vi "basic - VL Receive.vi"() -> ()   [LabVIEW 2020]
uses:
  _controls/comm_computedMAC-IP.ctl
  _controls/comm_verification_rx.ctl
  _controls/comm_udp_rx.ctl
  <extravilib>/ChannelInstances/Tag-bool/Write With Abort.vi
  <extravilib>/ChannelInstances/Tag-bool/Read With Abort.vi
  _polimorphicInstances/session/Fdx Create Session (Rx-VL-Oriented).vi
  bsp/AFDX_Receive/Fdx Create Rx VL.vi
  _polimorphicInstances/udpPort/Fdx Create UDP Port (RX-CommPort).vi
  _polimorphicInstances/control/Fdx Start (Rx).vi
  <extravilib>/ChannelInstances/Tag-bool/Instantiate.vi
  <extravilib>/ChannelInstances/Tag-bool/EndpointRead.vi
  <extravilib>/ChannelInstances/Tag-bool/Endpoint.vi
  _polimorphicInstances/control/Fdx Stop (Rx).vi
  _polimorphicInstances/session/Fdx Close Session (Port).vi
  AIM664LV.lvlib
  <extravilib>/ChannelInstances/Tag-bool.lvlib
panel:
  in  "DefaultPayloadMode (Full)":u32(ring) items=["FDX_PAYLOAD_FULL", "FDX_PAYLOAD_IP_EXT", "FDX_PAYLOAD_IP", "FDX_PAYLOAD_MAC"]
  in  "Board":u32
  in  "Port":u32=1
  out "CommPort Addresses":T1[](array[typedef])=[{"MACsrc"=[], "IPsrc"="10.1.33.1", "IPdest"="224.224.0.60"}, {"MACsrc"=[], "IPsrc"="10.1.33.1", "IPdest"="224.224.0.60"}] {"MACsrc" format="%.0x"}
  in  "VL Config":T2={"VlId"=60, "VLRange"=2, "VerificationMode"=0, "Bag"=0, "Jitter"=0, "MaxFrameLength"=0, "MaxSkew"=0, "VLBufSize"=32768, "FilterMode"=0, "FilterPosition"=0, "Padding"=0, "FilterMask"=0, "FilterData"=0, "MinFrameLength"=0} {"FilterMode" items=["FDX_RX_VL_FLT_DIS", "FDX_RX_VL_FLT_ENA ", "FDX_RX_VL_FLT_ENA_INV"]; "MaxFrameLength" format="%.0x"; "VerificationMode" items=["FDX_RX_VL_CHECK_ENA_DEFAULT"=65535, "FDX_RX_VL_CHECK_REDMAM"=16, "DX_RX_VL_CHECK_TRAFIC"=8, "FDX_RX_VL_CHECK_FRAMESIZE"=4, "FDX_RX_VL_CHECK_SNINTEG"=2, "FDX_RX_VL_CHECK_INVPAC"=1, "FDX_RX_VL_CHECK_DISA"=0]}
  in  "CommPort Config":T3[](array[typedef])=[{"PortType"=enum."FDX_UDP_SAMPLING", "SubVIId"=1, "domainID"=1, "sideID"=1, "locationID"=1, "partitionID"=1, "UdpSrcPort"=1, "UdpDstPort"=1, "UdpNumBufMessages"=1, "UdpMaxMessageSize"=1000, "UdpSamplingRate"=0}, {"PortType"=enum."FDX_UDP_SAMPLING", "SubVIId"=2, "domainID"=1, "sideID"=1, "locationID"=1, "partitionID"=1, "UdpSrcPort"=2, "UdpDstPort"=2, "UdpNumBufMessages"=1, "UdpMaxMessageSize"=1000, "UdpSamplingRate"=0}] {"partitionID" format="%.0b"}
  out "read time uS":u32(graph)=3177
  in  "poll rate mS 1":u32=10
  out "data":cluster{"Data":u8[]}[](array[cluster])
  out "BytesRead":u32[](array[numeric])
  out "current time":timestamp=timestamp(3686488955.9671674 s since 1904-01-01)
  out "current irig time":T4={"SignOut"=-1509901600, "DayOut"=16, "HourOut"=8, "MinOut"=7, "SecondOut"=53, "MilliSecOut"=368, "MicroSecOut"=508, "NanoSecOut"=600, "InfoOut"=0, "Mode"=3}
  in  "stop":bool
  out "PortInitOut":T5={"PortConfig"=0, "PortUsed"=1, "GlobalMemFree"=0, "SharedMemFree"=0} {"PortConfig" items=["FDX_SINGLE", "FDX_REDUNDANT"]}
  out "error out":errorcluster
  # "ARINC 664 - Receiving through VL (Virtual Link)"
  # "Overview: Setup the board to transmit package as raw frames.\nRequirement: One AIM ARINC-664 board with installed AIM ARINC 664 BSP.\nRestrictions: None.\nInstruction:\n1. Select the Board ID (0 if you have only one board in your system) and the port number. If you want to validate between two ports in one device, you can use tx board and Rx Board\n2. Run the VI.\n3. See the result in Current IRIG Time"
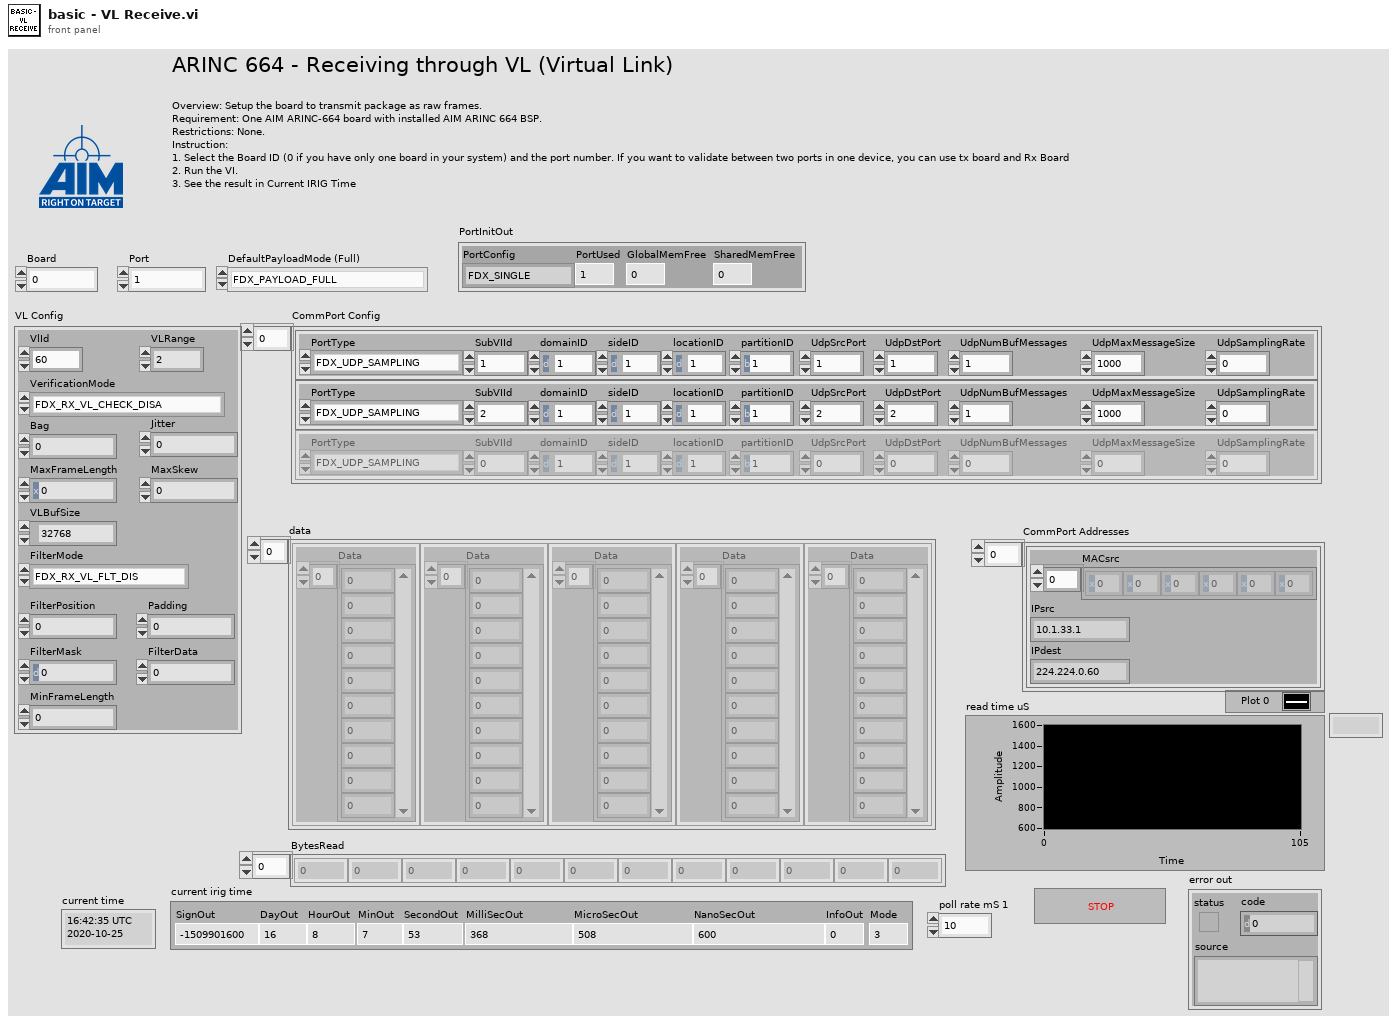
[diagram p1: front panel]
types:
  T1 = typedef "AIM664LV.lvlib/comm_computedMAC-IP.ctl" = cluster{"MACsrc":u8[], "IPsrc":string, "IPdest":string}
  T2 = typedef "AIM664LV.lvlib/comm_verification_rx.ctl" = cluster{"VlId":u16, "VLRange":u32, "VerificationMode":u32, "Bag":u32, "Jitter":u32, "MaxFrameLength":u32, "MaxSkew":u32, "VLBufSize":u32, "FilterMode":u32, "FilterPosition":u32, "Padding":u32, "FilterMask":u32, "FilterData":u32, "MinFrameLength":u32}
  T3 = typedef "AIM664LV.lvlib/comm_udp_rx.ctl" = cluster{"PortType":enum16{"FDX_UDP_SAMPLING", "FDX_UDP_QUEUING"}, "SubVIId":u32, "domainID":u8, "sideID":u8, "locationID":u8, "partitionID":u8, "UdpSrcPort":u16, "UdpDstPort":u16, "UdpNumBufMessages":u32, "UdpMaxMessageSize":u32, "UdpSamplingRate":u32}
  T4 = cluster{"SignOut":i32, "DayOut":u32, "HourOut":u32, "MinOut":u32, "SecondOut":u32, "MilliSecOut":u32, "MicroSecOut":u32, "NanoSecOut":u32, "InfoOut":u32, "Mode":u32}
  T5 = cluster{"PortConfig":u32, "PortUsed":u32, "GlobalMemFree":u32, "SharedMemFree":u32}
  T6 = typedef "Tag-bool.lvlib/))Channel.ctl" = refnum<queue>
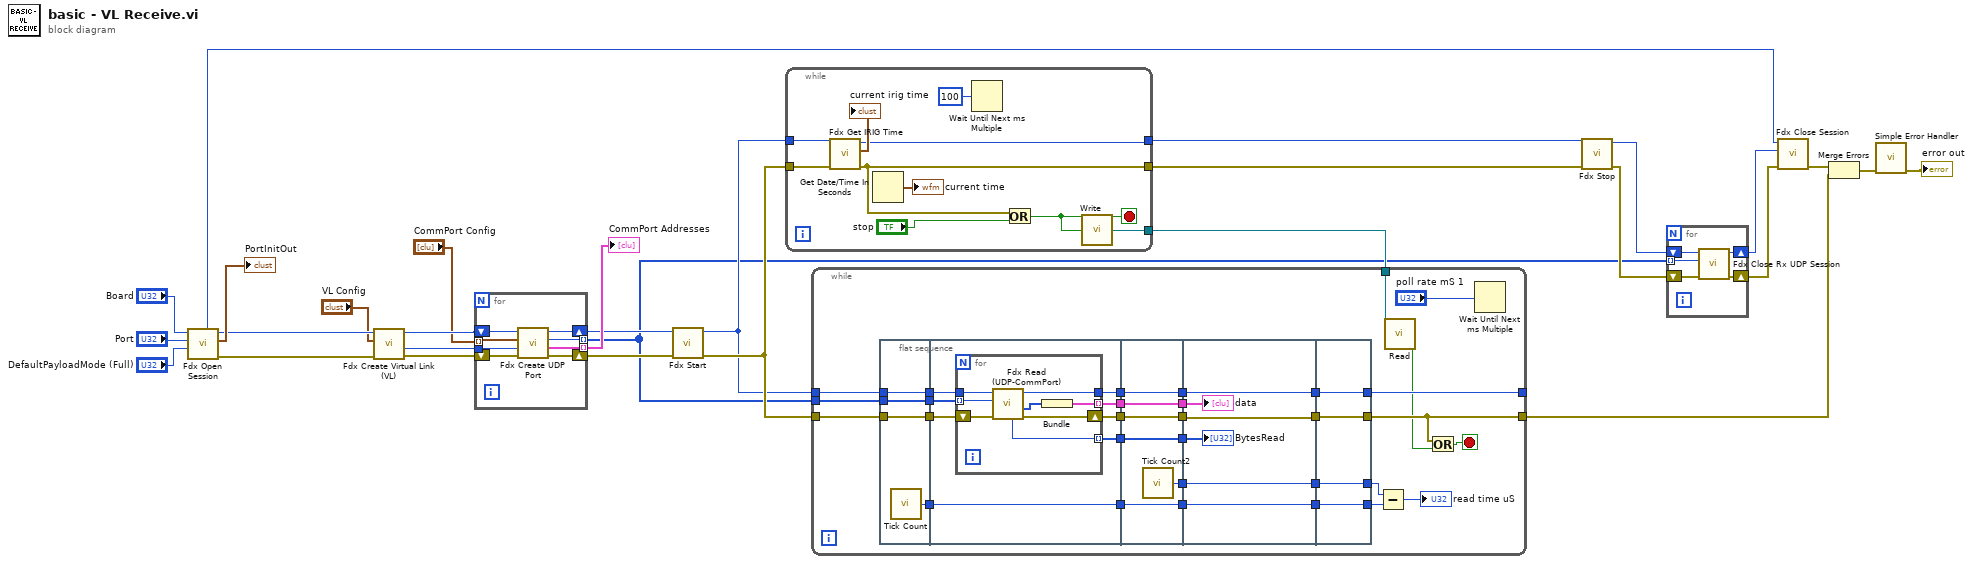
[diagram p0: block diagram]
diagram:
  n1 = call-poly "Fdx Open Session.vi"("DefaultPayloadMode (Full)"="DefaultPayloadMode (Full)", "port"="Port", "board"="Board") -> ("error out"=w14:errorcluster, "PortInitOut"=→"PortInitOut":T5, "InstrumentHandle_port out"=w15:u32, "InstrumentHandle_board out"=w3:u32)  [unwired: 3 in, 2 out]
  n2 = call-poly "Fdx Create Virtual Link (VL).vi"("error in (no error)"=w14, "VL Config"="VL Config", "InstrumentHandle_port in"=w15) -> ("error out"=w11:errorcluster, "VlId"=w10:u16, "InstrumentHandle_port out"=w12:u32)  [unwired: 6 in]
  n3 = for {
    tunnel: [w36] -> w28 mode=indexing
    tunnel: [w32] -> w4 mode=indexing
    shift-right: [w37] -> w29
    shift-left: w11 -> [w34]
    shift-right: [w35] -> w27
    shift-left: w12 -> [w33]
    tunnel: w10 -> [w31]
    tunnel: "CommPort Config" -> [w30] mode=indexing
    n4 = call-poly "Fdx Create UDP Port.vi"("error in"=w34, "VlId"=w31, "CommPort Config"=w30, "port handle in"=w33) -> ("error out"=w37:errorcluster, "computedAddresses"=w36:T1, "commPort handle out"=w32:u32, "port handle out"=w35:u32)  [unwired: 4 in]
  }
  "CommPort Addresses" <- w28
  n5 = call-poly "Fdx Start.vi"("error in"=w29, "InstrumentHandle_port in"=w27) -> ("error out"=w20:errorcluster, "InstrumentHandle_port out"=w5:u32)  [unwired: 8 in]
  n6 = while {
    tunnel: w5 -> [w46]
    tunnel: w20 -> [w45]
    tunnel: [w43] -> w23
    tunnel: [w42] -> w22
    tunnel: [w38] -> w18
    stop <- w39 stop-if-true
    n7 = call "Fdx Get IRIG Time.vi"("error in (no error)"=w45, "InstrumentHandle_board in"=w46) -> ("error out"=w42:errorcluster, "Curent Irig Time"=→"current irig time":T4, "InstrumentHandle_board out"=w43:u32)  [unwired: 7 in]
    n8 = Get Date/Time In Seconds() -> (seconds since 1Jan1904=→"current time":timestamp)
    n9 = Wait Until Next ms Multiple(millisecond multiple=u32 100) -> ()  [unwired: 1 out]
    n10 = Or(x=w42, y="stop") -> (x .or. y?=w39:bool)
    n11 = call <extravilib>:"Write.vi"("element"=w39) -> ("channel"=w38:T6)  [unwired: 1 out]
  }
  n12 = while {
    tunnel: w20 -> [w77]
    tunnel: w4 -> [w76]
    tunnel: [w64] -> _
    tunnel: [w57] -> w16
    tunnel: w18 -> [w52]
    tunnel: w5 -> [w49]
    stop <- w78 stop-if-true
    n13 = flat-sequence {
      tunnel: w77 -> [w81]
      tunnel: w76 -> [w82]
      tunnel: [w82] -> w72
      tunnel: [w81] -> w71
      tunnel: [w80] -> w70
      tunnel: w49 -> [w79]
      tunnel: [w79] -> w48
      tunnel: w72 -> [w84]
      tunnel: w71 -> [w90]
      tunnel: w70 -> [w89]
      tunnel: [w89] -> w69
      tunnel: [w88] -> w61
      tunnel: [w87] -> w58
      tunnel: [w86] -> w55
      tunnel: [w85] -> w53
      tunnel: w48 -> [w83]
      tunnel: w69 -> [w104]
      tunnel: [w104] -> w68
      tunnel: [w103] -> w65
      tunnel: [w102] -> w62
      tunnel: w61 -> [w102]
      tunnel: [w101] -> w59
      tunnel: w58 -> [w101]
      tunnel: [w100] -> w56
      tunnel: w55 -> [w100]
      tunnel: [w99] -> w54
      tunnel: w53 -> [w99]
      tunnel: w68 -> [w110]
      tunnel: [w110] -> w74
      tunnel: [w109] -> w66
      tunnel: w65 -> [w109]
      tunnel: [w108] -> w63
      tunnel: w62 -> [w108]
      tunnel: [w107] -> w60
      tunnel: w59 -> [w107]
      tunnel: w56 -> [w105]
      tunnel: w54 -> [w106]
      tunnel: [w114] -> w75
      tunnel: w74 -> [w114]
      tunnel: [w113] -> w67
      tunnel: w66 -> [w113]
      tunnel: [w112] -> w64
      tunnel: w63 -> [w112]
      tunnel: [w111] -> w57
      tunnel: w60 -> [w111]
      frame #0 {
        n14 = call "Tick Count"() -> ("Tick Count(uSec)"=w80:u32)
      }
      frame #1 {
        n15 = for {
          tunnel: [w97] -> w88
          tunnel: [w91] -> w86 mode=indexing
          tunnel: [w95] -> w85 mode=indexing
          tunnel: w84 -> [w94] mode=indexing
          tunnel: w83 -> [w93]
          shift-right: [w96] -> w87
          shift-left: w90 -> [w98]
          n16 = call "Fdx Read (UDP-CommPort).vi"("error in"=w98, "UdpHandle"=w94, "InstrumentHandle_port"=w93) -> ("error out"=w96:errorcluster, "ReadBuffer"=w92:u8[], "InstrumentHandle_port"=w97:u32, "MsgRead"=w95:u32)  [unwired: 4 in, 1 out]
          n17 = Bundle("ReadBuffer"=w92) -> (w91:cluster{"ReadBuffer":u8[]})  [unwired: 1 in]
        }
      }
      frame #2 {
        n18 = call "Tick Count2"() -> ("Tick Count(uSec)"=w103:u32)
      }
      frame #3 {
        "BytesRead" <- w106
        "data" <- w105
      }
      frame #4 {
      }
    }
    n19 = Subtract(x=w67, y=w75) -> (x-y=→"read time uS":u32)
    n20 = call <extravilib>:"Read.vi"("channel"=w52) -> ("element"=w51:bool)  [unwired: 1 in, 1 out]
    n21 = Or(x=w57, y=w51) -> (x .or. y?=w78:bool)
    n22 = Wait Until Next ms Multiple(millisecond multiple="poll rate mS 1") -> ()  [unwired: 1 out]
  }
  n23 = call-poly "Fdx Stop.vi"("error in"=w22, "InstrumentHandle_port in"=w23) -> ("error out"=w21:errorcluster, "InstrumentHandle_port out"=w7:u32)  [unwired: 8 in]
  n24 = for {
    tunnel: w4 -> [w115] mode=indexing
    shift-right: [w118] -> w19
    shift-left: w21 -> [w119]
    shift-right: [w116] -> w6
    shift-left: w7 -> [w117]
    n25 = call "Fdx Close Rx UDP Session.vi"("error in"=w119, "UdpHandle"=w115, "InstrumentHandle_port"=w117) -> ("error out"=w118:errorcluster, "InstrumentHandle_port"=w116:u32)  [unwired: 7 in]
  }
  n26 = call-poly "Fdx Close Session.vi"("error in"=w19, "InstrumentHandle_port in"=w6, "InstrumentHandle_board in"=w3) -> ("error out"=w17:errorcluster)  [unwired: 8 in]
  n27 = Merge Errors(w17, w16) -> (w2:errorcluster)
  n28 = call <vilib>:"Simple Error Handler.vi"("error in (no error)"=w2) -> ("error out"=→"error out":errorcluster)  [unwired: 4 in, 4 out]
